vi "FFT_Data_Processing.vi"() -> ()   [LabVIEW 2014]
uses:
  <vilib>/Analysis/baseanly.llb/Mean (DBL).vi
  <vilib>/Analysis/2dsp.llb/Power Spectrum (DBL).vi
  <vilib>/Analysis/2dsp.llb/1D Auto Correlation (DBL).vi
  <vilib>/Analysis/2dsp.llb/Real FFT.vi
  <vilib>/Analysis/2dsp.llb/Cross Power (DBL).vi
  <vilib>/Analysis/2dsp.llb/1D Cross Correlation (DBL).vi
  <vilib>/imath/engines/lvmath2/RunTimeEngine/BuiltInFunctions/win_hamming/NIMS_win_hamming.vi
  <vilib>/imath/engines/lvmath2/RunTimeEngine/BuiltInFunctions/coherence_ms/NIMS_coherence_ms().vi
  <instcachedir>/0/NIMS_coherence_ms()_BC56CBD83C8F45CD8D3E853BABAA39DC.lvgen/NIMS_coherence_ms()_BC56CBD83C8F45CD8D3E853BABAA39DC_000.vi
  <vilib>/imath/engines/lvmath2/RunTimeEngine/ErrorHandling/NIMS_Create Error From Enums.vi
  <vilib>/imath/engines/lvmath2/RunTimeEngine/NodeEndStatement/NIMS_NodeEndStatement_Output.vi
  <instcachedir>/0/NIMS_NodeEndStatement_Output_53EC0D466D134D7ABD903AC30B43404B.lvgen/NIMS_NodeEndStatement_Output_53EC0D466D134D7ABD903AC30B43404B_005.vi
  <vilib>/imath/engines/lvmath2/RunTimeEngine/ErrorHandling/NIMS_Finalize Error.vi
  <vilib>/ptbypt/Signal Generation.llb/Gaussian White Noise PtByPt.vi
  <vilib>/ptbypt/NI_PtbyPt.lvlib
  <vilib>/Simulation/ContinuousLinear/Implementation/NILVSim Transfer Function.llb/SIM Transfer Function (SISO).vi
  <vilib>/Simulation/Implementation/XNodeFramework/SimXNode/SimX.xnode
  <vilib>/Simulation/SignalDisplay/Implementation/NILVSim Time Waveform.llb/SIM Time Waveform (scalar).vi
  <vilib>/Simulation/DataSources/Implementation/NILVSim Pulse Generator.llb/SIM Pulse Generator (scalar).vi
  <vilib>/Simulation/Implementation/Shared/SIMSCR Execution Mode.ctl
  <vilib>/Simulation/Scripting/Companion Diagram/SimConfigNode/_simSolvers.ctl
  <vilib>/Simulation/Scripting/Companion Diagram/SimConfigNode/SimParams.ctl
  <vilib>/Simulation/Scripting/Companion Diagram/SimConfigNode/SimDog.xnode
  <vilib>/Analysis/NI_AALPro.lvlib
  <vilib>/Simulation/Implementation/Shared/SIM Bundle Sim Info.vi
  <vilib>/Simulation/Implementation/Shared/SIM Unbundle Sim Info.vi
  <vilib>/Simulation/Implementation/Shared/NILVSim_FinalizeModel.vi
  <vilib>/Simulation/Implementation/Shared/NILVSim_GetModelError.vi
  <vilib>/Simulation/Implementation/Shared/NILVSim_Initialize.vi
  <vilib>/Simulation/Utility/Implementation/NILVSim Get Time and IsAcceptedStep.vi
  <vilib>/Simulation/Implementation/Shared/NILVSim_Manager.vi
  <vilib>/Simulation/Implementation/Shared/NI_SIM_Implementation.lvlib
  <vilib>/Simulation/Implementation/Shared/NILVSIM_BeginStep.vi
  <vilib>/Simulation/Param Hierarchy/Typedefs/SIMPH Param Control Actions.ctl
  <vilib>/Simulation/Implementation/Shared/NILVSim_ParamChanged.vi
  <vilib>/Utility/error.llb/Clear Errors.vi
  <vilib>/Simulation/Implementation/Shared/SIMSH Read Queue.vi
  <vilib>/Simulation/ContinuousLinear/Implementation/NILVSim Transfer Function.llb/SIM Transfer Function Collector (SISO).vi
  <vilib>/Simulation/ContinuousLinear/Implementation/NILVSim Transfer Function.llb/SIM Transfer Function Distributor (SISO).vi
  <vilib>/Analysis/NI_AALBase.lvlib
panel:
  out "XY Graph":cluster{"X":dbl, "Y":dbl}[](graph)
  out "Coherence":cluster{"f0":dbl, "df":dbl, "magnitude":dbl[]}(graph)={"f0"=0.0, "df"=5.029169181251257, "magnitude"=array[24855 elements]}
  out "size(s)":i32=24856
  in  "INA Resistance":dbl=1000.0
  out "array":dbl[][](array[numeric])
  in  "file path (use dialog)":path=path "D:/Academic_Gaduate/Course/2016 Spring/2.131/Project/MyRIO/DAQ and Actuation DIO Stochastic Double Input 125kHz differential measurement and system ID with Bode Plot Analysis/04212016/RC/BinaryStochastic/042116_RC_Stochastic_4.csv"
  out "Phase spectrum":cluster{"f0":dbl, "df":dbl, "phase":dbl[]}(graph)={"f0"=0.0, "df"=5.029169181251257, "phase"=array[24855 elements]}
  out "Amplitude spectrum":cluster{"f0":dbl, "df":dbl, "magnitude":dbl[]}(graph)={"f0"=0.0, "df"=5.029169181251257, "magnitude"=array[24855 elements]}
  in  "Sample_Frequency (Hz)":dbl=125000.0
  out "Waveform Chart":waveform(dbl)(graph)={"t0"=timestamp(0.01 s since 1904-01-01), "dt"=1.0, "Y"=[1.8810764409104788]}
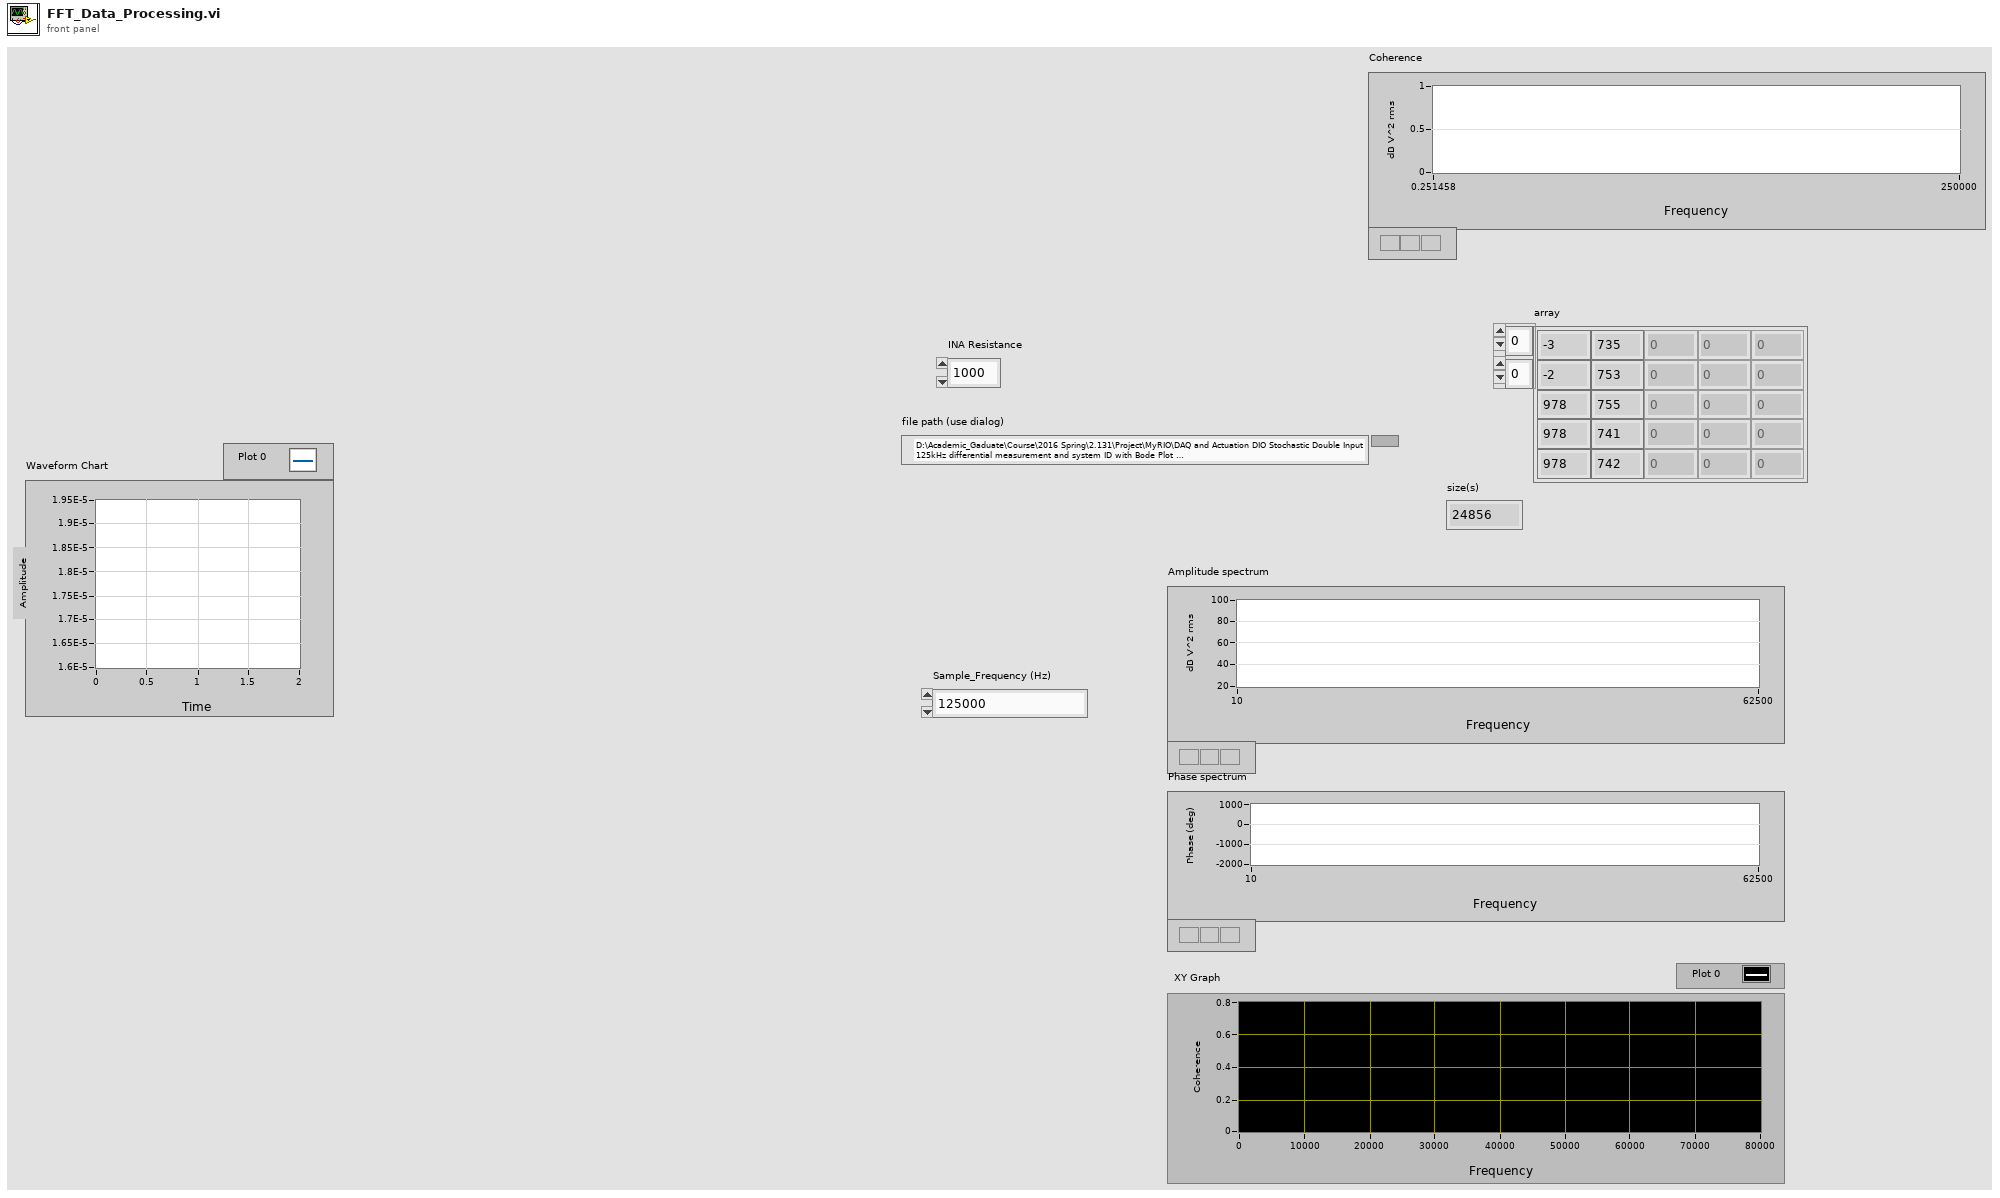
[diagram p1: front panel]
types:
  T1 = enum16{"open", "replace", "create", "open or create", "replace or create", "replace or create with confirmation"}
  T2 = typedef "SIMSCR Execution Mode.ctl" = enum16{"Simulate to Completion", "Single Time-Step Simulation (Fixed Step Only)"}
  T3 = typedef "SIMPH Param Control Actions.ctl" = enum16{"get params", "set params"}
  T4 = typedef "SimParams.ctl" = cluster{"Initial Time (s)":dbl, "Final Time (s)":dbl, "Step Size (s)":dbl, "ODE Solver":T5, "Minimum Step Size (s)":dbl, "Maximum Step Size (s)":dbl, "Relative Tolerance":dbl, "Absolute Tolerance":dbl, "Software Timing":bool, "Initial Step Size (s)":dbl, "Automatic Fixed Step Size?":bool, "Automatic Discrete Step Size?":bool, "Discrete Step Size (s)":dbl, "Calculate using Time Step":bool, "Solver Wired?":bool, "Prev.Frm.Expected End":u64, "Prev.Frm.Actual End":u64, "Prev.Frm.Finished Late?":bool, "Prev.Iter.Expected End":u64, "Prev.Iter.Actual End":u64, "Prev.Iter.Finished Late?":bool, "Expected Iteration Start":u64, "Actual Iteration Start":u64, "Expected Frame Start":u64, "Actual Frame Start":u64, "Source Name":string, "Name":string, "Period":i64, "Deadline":i64, "Offset":i64, "Start":i64, "Priority":i32, "Timeout":i32, "Processor":i32, "Mode":enum32{"No Change", "Process missed periods, maintain original phase", "Discard missed periods, maintain original phase", "Process missed periods, ignore original phase", "Discard missed periods, ignore original phase"}, "Wakeup reason":enum32{"Normal", "Aborted", "Asynchronous wakeup", "Timing source error", "Timed loop error", "Timeout"}, "Error":errorcluster, "Source Type":string, "Secondary Source Type":string, "Global End Time":u64, "Global Start Time":u64, "Full Solver Reset":bool, "Execution Mode":T2, "Nan/Inf Check":bool, "Custom Solver Library":string, "Solver Is Variable":bool, "custom solver name":string, "Signal Collection Decimation":u32}
  T5 = typedef "_simSolvers.ctl" = enum16{"Runge-Kutta 1 (Euler)", "Runge-Kutta 2", "Runge-Kutta 3", "Runge-Kutta 4", "Runge-Kutta 23 (variable)", "Runge-Kutta 45 (variable)", "BDF (variable)", "Adams-Moulton (variable)", "Rosenbrock (variable)", "Discrete States Only", "SDIRK 4 (variable)", "Radau 5 (variable)", "Radau 9 (variable)", "Radau 13 (variable)", "Radau [Variable Order] (variable)", "Gear's Method (variable)", "Linearizer", "State Query", "Trim Eval", "Custom Solver"}
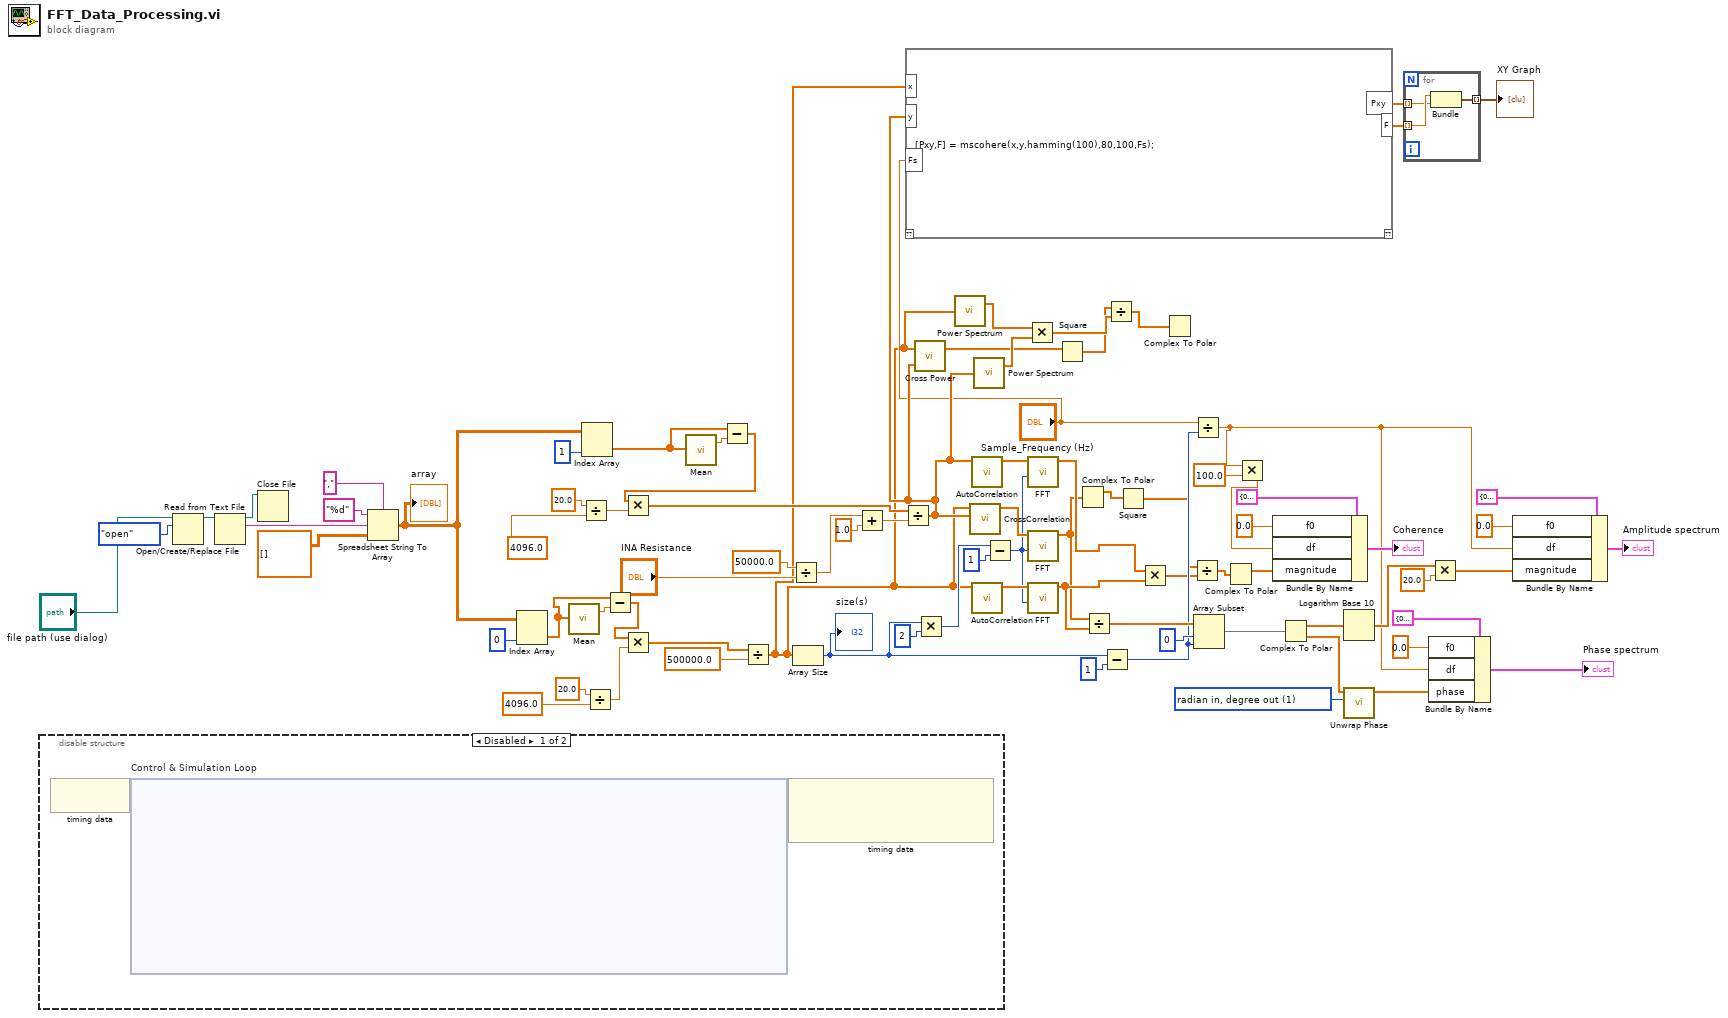
[diagram p0: block diagram]
diagram:
  w39 = 1 items=["radian in, radian out", "radian in, degree out", "degree in, degree out", "degree in, radian out"] ("phase unit")
  n1 = disable-structure shown="Disabled" {
    frame Disabled {
      n2 = node-c288() -> (w85:variant)  [unwired: 1 in]
      n3 = node-c254 "Control & Simulation Loop"(w85) -> (w84:variant)
      n4 = node-c288(w84) -> ()  [unwired: 3 out]
    }
    frame Enabled {
    }
  }
  n5 = Open/Create/Replace File(file path (use dialog)="file path (use dialog)", operation (0:open)=T1."open") -> (refnum out=w81:refnum<file>)  [unwired: 4 in, 2 out]
  n6 = Read from Text File(file (use dialog)=w81) -> (refnum out=w76:refnum<file>, text=w79:string)  [unwired: 3 in, 2 out]
  n7 = Close File(refnum=w76) -> ()  [unwired: 1 in, 2 out]
  n8 = Spreadsheet String To Array(delimiter (Tab)=",", format string="%d", spreadsheet string=w79, array type (2D Dbl)=dbl[][] []) -> (array=w23:dbl[][])
  "array" <- w23
  n9 = Index Array(array=w23, index (col)=0 ("disabled index (col)")) -> (element=w19:dbl[])  [unwired: 1 in]
  n10 = call-poly <vilib>:"Mean.vi"("X"=w19) -> ("mean"=w20:dbl)  [unwired: 1 out]
  n11 = Divide(x=20.0, y=4096.0) -> (x/y=w52:dbl)
  n12 = Index Array(array=w23, index (col)=1 ("disabled index (col)")) -> (element=w22:dbl[])  [unwired: 1 in]
  n13 = Divide(x=20.0, y=4096.0) -> (x/y=w45:dbl)
  n14 = Subtract(x=w19, y=w20) -> (x-y=w18:dbl[])
  n15 = Multiply(x=w18, y=w45) -> (x*y=w31:dbl[])
  n16 = call-poly <vilib>:"Mean.vi"("X"=w22) -> ("mean"=w21:dbl)  [unwired: 1 out]
  n17 = Subtract(x=w22, y=w21) -> (x-y=w17:dbl[])
  n18 = Multiply(x=w17, y=w52) -> (x*y=w30:dbl[])
  n19 = Divide(x=w31, y=500000.0 ("x")) -> (x/y=w8:dbl[])
  n20 = Divide(x=50000.0, y="INA Resistance") -> (x/y=w50:dbl)
  n21 = Array Size(array=w8) -> (size(s)=w61:i32)
  "size(s)" <- w61
  n22 = Add(x=w50, y=1.0) -> (x+y=w41:dbl)
  n23 = Divide(x=w30, y=w41) -> (x/y=w10:dbl[])
  n24 = mathscript code="[Pxy,F] = mscohere(x,y,hamming(100),80,100,Fs);"("x"=w8, "y"=w10, "Fs"="Sample_Frequency (Hz)") -> ("Pxy"=w1:dbl[], "F"=w2:dbl[])  [unwired: 1 in, 1 out]
  n25 = call-poly <vilib>:"Cross Power.vi"("Y"=w10, "X"=w8) -> ("Sxy"=w11:cdb[])  [unwired: 1 out]
  n26 = Multiply(x=w61, y=2) -> (x*y=w72:i32)
  n27 = call-poly <vilib>:"Power Spectrum.vi"("X"=w8) -> ("Power Spectrum"=w16:dbl[])  [unwired: 1 out]
  n28 = call-poly <vilib>:"CrossCorrelation.vi"("Y"=w10, "X"=w8) -> ("Rxy"=w74:dbl[])  [unwired: 8 in, 1 out]
  n29 = call-poly <vilib>:"AutoCorrelation.vi"("X"=w10) -> ("Rxx"=w37:dbl[])  [unwired: 9 in, 1 out]
  n30 = call-poly <vilib>:"AutoCorrelation.vi"("X"=w8) -> ("Rxx"=w75:dbl[])  [unwired: 9 in, 1 out]
  n31 = call-poly <vilib>:"Power Spectrum.vi"("X"=w10) -> ("Power Spectrum"=w15:dbl[])  [unwired: 1 out]
  n32 = Subtract(x=w72, y=1) -> (x-y=w36:i32)
  n33 = Multiply(x=w16, y=w15) -> (x*y=w14:dbl[])
  n34 = call-poly <vilib>:"FFT.vi"("FFT size"=w36, "X"=w37) -> ("FFT {X}"=w27:cdb[])  [unwired: 8 in, 1 out]
  n35 = call-poly <vilib>:"FFT.vi"("FFT size"=w36, "X"=w74) -> ("FFT {X}"=w24:cdb[])  [unwired: 8 in, 1 out]
  n36 = call-poly <vilib>:"FFT.vi"("FFT size"=w36, "X"=w75) -> ("FFT {X}"=w26:cdb[])  [unwired: 8 in, 1 out]
  n37 = Square(x=w11) -> (x^2=w12:cdb[])
  n38 = Complex To Polar(r * e^(i*theta)=w24) -> (r=w25:dbl[])  [unwired: 1 out]
  n39 = Divide(x=w24, y=w26) -> (x/y=w63:cdb[])
  n40 = Subtract(x=w61, y=1) -> (x-y=w58:i32)
  n41 = Divide(x=w12, y=w14) -> (x/y=w13:cdb[])
  n42 = Square(x=w25) -> (x^2=w28:dbl[])
  n43 = Multiply(x=w27, y=w26) -> (x*y=w33:cdb[])
  n44 = Complex To Polar(r * e^(i*theta)=w13) -> ()  [unwired: 2 out]
  n45 = Divide(x=w28, y=w33) -> (x/y=w29:cdb[])
  n46 = Divide(x="Sample_Frequency (Hz)", y=w58) -> (x/y=w7:dbl)
  n47 = Array Subset(array=w63, index=0, length=w58) -> (w64:cdb[])
  n48 = Complex To Polar(r * e^(i*theta)=w29) -> (r=w4:dbl[])  [unwired: 1 out]
  n49 = Multiply(x=w7, y=100.0) -> (x*y=w5:dbl)
  n50 = Bundle By Name(cluster=cluster{"f0":dbl, "df":dbl, "magnitude":dbl[]} {"f0"=0.0, "df"=0.0, "magnitude"=[]} ("Amplitude spectrum"), "f0"=0.0, "df"=w5, "magnitude"=w4) -> (→"Coherence":cluster{"f0":dbl, "df":dbl, "magnitude":dbl[]})
  n51 = Complex To Polar(r * e^(i*theta)=w64) -> (r=w60:dbl[], theta=w38:dbl[])
  n52 = Logarithm Base 10(1:w60) -> (0:w68:dbl[])
  n53 = call <vilib>:"Unwrap Phase.vi"("phase unit"=w39, "Phase"=w38) -> ("Unwrapped Phase"=w40:dbl[])  [unwired: 8 in, 1 out]
  n54 = for {
    tunnel: w2 -> [w406] mode=indexing
    tunnel: w1 -> [w405] mode=indexing
    tunnel: [w404] -> w3 mode=indexing
    n55 = Bundle(w406, w405) -> (w404:cluster{dbl, dbl})  [unwired: 1 in]
  }
  "XY Graph" <- w3
  n56 = Bundle By Name(cluster=cluster{"f0":dbl, "df":dbl, "phase":dbl[]} {"f0"=0.0, "df"=0.0, "phase"=[0.0, -31.46771497568485, -28.75800712836132, -41.40521112388251, -28.23254003958854, -10.307643755414622, -48.402035704012796, -54.988080356169355, -6.260155572788149, -114.48865953158258, 8.840814305252367, -81.75181328535328, 2.5045447437835056, -4.4432479279741095, -91.23410525561975, 31.80581741631602, -114.44832858997734, -27.80131859077831, -99.25569904439564, -30.088844331129934, -103.06596414735802, -66.66233183584428, 12.455917853016478, 109.28759197945335, -66.14168263333863, -144.83425351569642, 51.71723004569318, -59.12936901186461, -59.94315211957277, -44.52651345174281, -83.39567725724885, -88.80210274367009, 173.64945828897015, -22.022991001879543, -176.90163746313618, -45.43423776031069, -174.56084625229602, 23.97985521334657, -111.39703590450088, -88.75411195664891, 17.490204367239716, -109.71720216205237, 15.903183296946878, -63.74675570783637, -76.38848380866358, 90.4171618729539, -67.70206212228267, 173.17746062348021, -63.34328741918001, 97.88702687250597, -26.830346465652713, -178.56862486837178, -28.233947423969404, -69.71520075870326, -93.38491152339505, 172.31861385368967, -24.72816138371724, -158.6603632884339, -63.92637331120567, 25.979182283576865, -176.178680883384, -54.992745526133994, 154.66292784768336, -21.75898247362432, 147.62448353052594, -48.4012168873971, 173.61513877249942, -91.40498135572582, -29.27842403446698, -90.12818047003235, 44.89492509568193, -85.02569711983062, -161.62807827258007, -30.33210234328775, -167.38943949322578, 17.714982838532073, 128.95801741205386, -67.90830100247624, 133.7770774630165, -28.626976629449626, -63.62310170383254, -117.87464062810677, 81.94531443559661, -93.09760124996781, 23.909644860719627, -101.32638644807278, -24.510873351315627, -168.41200063244855, -72.35935696130369, -155.28973739698282, -17.847314598481347, 78.21905993530349, -75.2179881300336, 158.254123483706, -113.64472897818374, -7.605633196806257, -179.31194749940937, -31.704382462216028, 176.59993683257554, -3.9100568867706125, -175.3215455037979, -37.06483139906273, -143.58448093876837, 20.571245493011833, -118.99832924113697, -96.78723400578556, -60.086953107243204, 122.97366891032519, -45.543749408235314, -91.64436597307613, 27.874487865472883, -44.86713542183372, -178.07594038380435, -86.92786166047328, 82.4094513217639, -78.34921684511612, -173.92693798878386, 102.4715615364932, -33.202770362216675, -119.88125106432467, 27.96070642572587, -143.51766607705275, -110.53171785865658, 14.030389804595977, -14.364430460296093, -121.02086313650614, 41.55311803721051, -82.14295365670695, 4.975296548772393, -146.7149096680376, -101.59304285295177, 29.849633712272396, -82.48816912553207, -149.48005476874508, 17.8777224533454, -153.22017067339883, -55.88267286162645, -73.12223389390026, -177.0689123580233, -101.71777995720713, -19.5987345915357, 48.39071628315272, -104.51560193133216, 106.24875412055499, -64.62181776044855, -152.49158868871936, 90.50578375571689, -110.23177544712142, 178.7743822962101, 8.933446493462752, -117.43777414097968, 33.78573575385322, 3.753644677644808, -133.54790142199468, 155.06753756966313, 1.313093243393488, -135.93501009935378, 102.88813110897146, -65.0985044001864, -22.667258074295468, 139.20059133429496, -50.73701255959797, 169.65584439562346, -4.395964236758193, -65.67336673335154, 95.38893308207317, -151.4067275831482, -135.1595759134875, -50.630333757584644, 86.38052475049209, -105.4818844884823, 48.68364954626779, -63.32067960398621, 152.87921036982615, 11.833828912216703, -14.298996026707998, -153.77260213733103, -43.14750001054217, 59.32361441752411, -131.55695844776793, -58.17994776721444, 70.44010783175709, -128.00748777563172, -68.53969421568672, -21.430548261334962, 132.6995122419159, -57.382207495062104, 104.60385375657543, 176.2681159822832, -12.528130482428411, -113.88004350080426, 6.718207285255911, -158.558628085825, -74.33498613287863, 83.3039064212861, -159.12090829011342, 10.554276562274639, -75.93691675536499, 53.72426810131386, -147.92326776688313, 42.16756652088333, -110.59744086394932, 13.00099316823571, 42.89530864726003, -78.5100056583534, -14.864119179247732, 151.771235214809, -53.33854934192464, -50.18504546090332, -78.10915320757155, 107.61492267174592, -41.731323391150696, -171.9549311336031, -31.909487386903535, -54.76941049884478, 161.99647147822193, -23.644807465324686, -139.42463002301935, 48.18016831507575, -137.63420984995042, 12.858622069483772, -144.83283655524738, -78.58801072388744, 56.23414488656744, -82.52800501693756, 165.1339518127335, 30.985754421181294, -50.87159030515992, -108.7703977965099, 104.96572974047947, -45.2937013625406, -108.84268401885568, 44.80515131574169, -139.81653610936894, -5.854579467043601, 139.24625549981425, -34.43047469570014, -130.57782005611404, -75.90546203446466, 76.71414237862456, -115.33869977557293, -152.1695207386769, 23.916191636708742, -157.80987721359594, -7.3317827307557675, 118.03670607456142, -122.24723240808913, 7.45872793350562, -40.91520539379452, 126.433151740827, -66.45542530364317, 111.57432009746935, -72.44942344083017, -177.4506210892957, -98.91073477511371, -7.729660477553103, 10.465818868467291, -85.6936671592382, -81.63472484446946, -142.59977661658678, 128.460132193279, -38.475073345298455, -67.30940359671469, 123.49482022783103, -97.1053140060935, 145.19216903060635, 19.599574149358055, 86.71319792618822, -59.42600601366192, 144.78547374608254, -0.14154390010495188, -31.99696885455758, -95.14990183095408, 17.55567657493523, -114.4051716245541, 123.83652692238601, -54.112354263827676, 111.56127409377314, -96.23472855569044, -164.82585042487696, -5.170563653506037, -152.92260427891915, -144.945554637376, 4.847235795070112, -119.10529254609949, 125.58380441248624, -63.22633423069135, 16.491596036524914, -169.19469396356925, -59.49742518985056, 99.33906473700418, -83.19230064604379, 94.70172496456746, -69.26753585553224, 93.20284400521376, -149.19174515783365, 32.644347404502724, -144.99653166541907, -5.748775767562918, 132.46944910894436, -70.188539813744, -175.15797843215728, -18.781631461778034, 139.2296455769892, -45.83812731645386, 159.7977626761071, -9.006363901405047, 148.21713714850534, -100.8278607774186, 55.930164359566405, -158.55075386155477, -103.64878607543045, -47.70206737703835, -65.34411503659574, 67.87094437951615, -154.64047195169766, 97.88783811393293, -5.57745461676379, -78.1709697035549, 78.52481788767172, 161.5334038052565, -109.8413047486903, 71.77211881090538, -4.575980521272304, -133.59202718799017, 61.733256861048496, 178.73417565413922, -47.53771825336581, 125.45827259728232, -97.1902841273301, 52.950131640632364, -154.25843315518011, 5.8136678258338845, -155.26807894125346, -51.157307142112785, 99.78819729052276, -48.97948721442834, 169.6472766422358, -117.99599455441421, 25.708792715303733, 131.97176948195855, -64.40284134065979, 111.90384579625118, -127.68827211261325, -77.79968188970696, 43.89611166074449, -160.45284620783127, 8.44734072748546, -149.78104520145075, -77.22735970987173, 159.98715516082572, -89.99063430205264, 45.70732002040879, -139.86300077763389, -6.566845107941335, 178.30876547862576, -22.561851211410573, 37.55133985052249, -149.05052759820148, -29.6953915669966, 95.88142220084387, -101.30091321782635, 23.223671482431147, -157.61569681073925, 32.07479172229752, -71.3688731058624, 2.5795540168955897, 120.05824105976018, -95.05769691572468, 37.51344432680482, -121.41122349093216, -142.04667587013134, 45.927259881274615, -134.5453172929541, 33.96968894493717, 153.058526546883, -140.03677728629194, 3.5646310942392696, -175.37291939786292, 14.115882878139795, -156.173477913963, -70.16579453905345, 91.56497193006136, -77.36117907923929, 59.233660597809425, -127.4719648111601, 56.51477730558104, -84.79620262857178, 86.58630420746188, -118.28259178761235, 22.600459669840806, 146.04464592728684, -77.89681873325401, -5.689349256760081, 177.24762803403777, -67.73763403578465, -1.8103440796276928, -115.0305743613975, 42.78528548717108, -106.57160168656428, 101.99012391694329, -102.41599801509702, 49.34066109247137, 178.44665732631697, -61.34206176169528, 132.87965238205607, -11.546056273837774, -125.65619450370565, 54.12229834647187, -127.60567202299247, 48.993493963204884, -16.604257356824057, -173.03075984094417, -47.372369968303495, 46.82445661446543, 68.31108839735339, 76.53022405615046, -159.4911598984052, 36.484166933763284, -47.776958039264834, 152.2068219538879, -69.4577862169963, 23.72800166288421, 151.48388845297458, -16.493785662288833, -171.7401814752173, -64.656079915525, -56.13125155943886, 82.01996288505002, -63.94387574731906, 124.71550967915313, -104.95295949349935, -67.38813885713685, 77.12067398170372, -101.33147779856687, 99.31134042143898, -64.55196472267788, -151.67999889218746, 113.13764572404774, -36.53419971497588, -134.1711272925018, 71.0322618140203, -163.46692161183003, -130.37776991970134, 58.37272802003515, -107.62472868622736, 92.95279272623449, -49.150748419198734, 159.36012917745043, 55.28737975676292, -110.16360848814493, -53.79860569519096, 104.49602190989943, 148.55577400818933, -30.020328942202788, -68.77381027418048, -42.15810867554653, 124.2170657880268, -86.95369614934374, 44.99512130882773, 177.32845100229312, -52.64196228170846, 46.20102763955148, -108.80445041232439, 62.10585572867235, -102.53934126921365, 145.9677583834663, -87.72193055370626, 7.430962421708717, 172.95218029826705, 4.4222030934162095, -131.33811798336814, 37.479163647581316, 137.83109311522614, -34.772558001913914, 152.95764683962005, -26.945111117281396, 166.68720416268573, -28.35898721082636, -102.96758495536596, 99.62582554177011, -81.23530180181987, 46.95581407891729, -125.39186806017632, 141.14774219662723, -65.91933405996008, 124.5369717528866, 112.16827006625896, -52.174323660626484, 130.56766513060325, -92.17901272631585, -99.80861309109997, -15.580125933333163, 178.68459291382678, 65.85001986602701, -85.62453959075624, 80.16771494845275, -63.09056610855369, -22.22041093173988, 142.374831558324, -22.723043570811264, 179.6131973929219, 1.0719245177840404, -88.1651047885446, 117.3162732148612, -60.235562901182256, -107.97892141496881, 162.13789603953347, 12.79775668263484, -159.941273163866, -112.3033138485895, -6.702876591119159, -175.53346605334087, -32.7521632120629, 148.57881181169574, -11.417752403481312, -169.89475358248, -33.20930187301011, 82.27334674193816, 172.04980593620093, -122.82110283025958, -42.916824763589396, 46.67338200369259, -155.2949042573867, -105.63553113653434, -107.62874242849799, 11.775202677368716, -171.23287115203678, -2.029325683277578, -162.5560667916255, 73.31010367618042, -107.93952835877826, -83.0493564353863, 52.09254527340971, -143.1028799072984, 53.765912683226226, -34.19495582188307, -117.75357133516779, 31.834257499681126, -140.93286631533525, 20.285152783977193, -162.04195864800806, 153.64371771682758, -73.66007185930609, 15.963436915003053, -171.21157098983684, -47.68895068390904, 66.4135578918687, 174.73664348470854, -46.579508638827356, 106.03859109730527, -109.91539448636465, 39.172417305631974, 145.77979102715958, -9.962680136496868, -164.42924385477494, -144.44561580277627, -69.78123459385885, -113.22071531978678, 1.218258742126064, 143.16141050902604, -157.77775989154455, -30.270285893319095, 166.15106846550387, -45.34197099655759, 137.05342066451018, 20.241780198571846, -102.77142543056473, 31.439785015283583, -121.94168892212197, 143.20819621702185, -19.50689927100417, -172.02714961369415, 14.333717594969812, -174.54550977736082, -38.23299518978718, -26.566119797522497, 145.54151457275842, -27.851441052904736, -163.1321157748263, 75.3014631451511, -94.74166019476999, 37.075911773395255, 155.54222543194072, -98.9395351512745, 148.13703747510186, -17.54789487058411, 143.79080232675827, -82.71301752835367, 71.3821044984081, -124.21247549991963, -1.6409856573868462, 19.6700330708455, 160.14775353560006, -16.49430253911016, -164.78180265396531, 12.760891558196134, -179.47420233424083, -5.793119973627547, 69.40140401989008, -85.35709611715286, 120.10014940793037, -104.09159686676787, 26.31025850963576, -83.18524249721266, -179.06877555105402, 71.26471876869424, -65.84400382413854, 19.518368314758515, 154.98160428075326, -39.27619259227029, 163.50923755813903, -50.03350589385845, -9.115898207634226, 130.84824117370394, -46.68826854993543, -148.71498865685814, -22.5834873291525, 132.6178627343492, -134.46027090254492, -2.8014924912677923, 2.4602588300456407, -20.736466264500084, -130.69158165429175, 150.66416663985305, -11.018068033122065, 171.6304217452683, -96.58990485321286, 77.83444641407394, -99.09283298242498, 88.80014570919934, -40.586998724210204, -35.179264249983795, 160.7340227956574, -6.810605241887145, -139.76389074792675, 61.4695137232016, 21.189936050034103, -98.82360269013745, 116.59527939088214, -8.355189026823824, 175.8100810017669, -8.629108482243616, -173.90491830172104, -79.85592225607972, 87.32016128248391, -91.81291748729721, -13.435477477820484, 96.50857130191405, -109.38180407495078, 33.06042963793669, 162.2011521762079, -117.94163565196628, -4.833287709282053, -62.12189719388706, 116.03937464806818, -57.917706915940535, 149.82527299038165, -51.82821745375959, 122.61039417676135, -44.556770160055926, -178.79931798390376, 73.21959964459208, -49.68220726056265, -88.4753258698242, 85.97647885149128, -38.29177733636641, -143.88884710240126, 5.282625504869, 141.10625269184, -57.50253327360124, 39.18691565225554, -159.6754196513465, -116.14617655830526, 95.22297266469835, -144.2484002418386, 28.899643887893554, -144.2272853862776, -37.74225611166511, 102.20586557689614, -59.82479773715672, 127.04189962515147, -46.24791124113113, 68.08629766481732, -156.7578294816097, -11.434921889037966, -162.7636201167861, 65.9875644978628, -34.46832773201904, -78.56948038746317, -6.341337929151649, -108.67685939124134, -106.89313197435935, 86.38952053728252, -82.93911771001973, 173.25389098385997, 67.40056048245822, -125.26619173900407, -37.805267152913395, -175.16220300153662, -140.71414280919208, 24.3021970024091, -150.81559287743767, 61.64820799188565, -135.28671942766917, 52.632055272904026, -89.42932587679499, 98.47854234743062, -39.87945695164611, -162.66519730541248, 11.68692118129435, -166.08307632599565, -88.98536844861681, 87.7653832187781, -59.430681173676724, 107.1788677654589, -87.82119051152033, 51.711884791693265, -178.07871544746556, 37.41838157670529, -55.35611367871979, -84.61570240600459, 94.65796995336078, -129.98746807541917, 58.335236715745765, -99.00946937428698, -27.388117599098656, 157.22388234666346, 72.24371871312997, -147.39896486209406, -132.6777473905325, -31.25385142571185, 74.26515240712175, -84.67039004635154, 94.80636631950513, -174.6516234468396, -170.3480501081504, -48.02777153805316, 51.75317164614029, -91.701517555401, 133.0172297974163, -7.30159849250651, -113.17171907810842, 44.91847253132216, -101.68955446502213, -112.83910396609542, 76.41050489240513, -96.71151005959905, 62.37966193166177, 174.59527102428734, -74.50503041737309, 102.74242740569944, -167.43185591844207, -28.974517625091067, 114.03751275726806, -52.52542778132872, 140.60970417095436, -43.560106659883395, 148.19389046654692, 62.03454906051373, -37.963677576846045, 154.55973613044287, 146.4805228355848, -16.955183383517827, 160.5658961892464, 41.884605965508264, -102.22531021640862, 66.33884226578459, 125.35537253171245, -93.07124847733196, 43.603115837203596, -35.825264703512545, -134.75332606919338, 140.3915945396924, -170.58539119057713, -4.3555387719877405, 166.02689974489226, -173.60083831016271, -0.12867793207221537, -164.76794171616692, 39.46321438891706, -71.26099387456847, 117.49796589596059, -32.12016123027836, 7.625896306543184, -151.83905484477293, -48.434939537281075, 53.64831087302935, -93.18411966205646, -98.36993493084799, 119.87917242870013, -108.55893117369165, -81.9910561163668, 95.0089679392402, -72.73671350427458, -14.702075420706603, 144.29025842674645, 3.0096227078141595, 174.39608030714825, -47.32134892884564, 130.1200593091527, 3.010297210957817, -149.96378770274794, 5.15648604979302, -131.00767475137724, -139.2648166197183, 51.05469049011057, 137.7627910319741, -129.56436731345153, -4.398610626420822, -128.85975701865624, 172.0314351621999, 19.536121307586072, -128.33535280968172, 115.03643800205525, -167.4008694494514, -99.78729461742101, 2.1618823895867507, 175.86714720509178, 27.870601656544217, -134.23437033976293, 61.752379570873074, -58.764272188723105, 140.50940594389758, 17.401790900348622, -76.88446792601037, 112.93800811739614, -74.47023687960714, 57.75177664789759, -135.33399721576845, -4.171499467230711, 158.58563404735605, 0.3753823843596019, -124.364687997409, -71.42039127455385, 89.7699642964547, -61.78524015886245, 139.76552443283884, -48.05344181609611, 172.2204000780463, 6.5441568360572555, -161.357014987678, -163.859193026889, 31.148918252059225, -74.63094220037475, 54.449483825565146, -141.07611084637665, -59.928523683736344, -111.59721137682088, 136.18591667878417, 51.20836380129699, -102.00998276251163, 69.38881272956878, -6.650584423835163, -119.84758918182608, -171.28476431719838, 31.745429699844387, -146.88562824741777, -41.455445941199955, 53.61648403891242, -83.30618114791412, 174.65974179855394, 98.65615679714519, -35.27670632618104, 94.2201132403794, -155.93415721486912, -6.581542390692745, -179.32672267917255, 175.13750093955665, -14.377608913808187, 148.30243299082807, -75.77067841132367, 38.9797740122615, -132.1587412992525, 106.49646205369946, 8.407250852124852, -35.496741621256454, -173.13138141404895, -15.555504023221577, -41.09548969322256, 103.51834305585722, -76.63858633555844, 83.08988233557466, -104.31389048078786, 152.10523290311446, 24.12399022599241, -111.12207877005906, 78.26259707356425, -112.02416060399644, 15.314106421968939, 101.82627173313676, -93.85166587574152, -78.05401638398496, 80.07712418944736, -124.77812823558038, 35.24366770793687, -175.3845889000318, -132.36572514301386, 40.5756213070226, -156.20187378885308, 171.9056817310974, -39.56045326497815, -168.07294285346202, 69.84033971188616, -128.70404232383888, 55.7018856169047, -106.91461481830608, 61.33433465707653, -79.25612475595284, 120.3157571372352, -31.727767728482117, -131.03860078296557, 52.30500145215631, -22.159778917101875, 47.784773735495726, -167.58098485630725, 61.19805538687596, -97.43659050196452, 172.61620968167725, 79.22607520811626, -95.95857423816624, 66.45261522120416, -84.99681059301679, 90.93092605365476, -109.87924739570839, 81.26444224879198, -48.34416826511803, -64.58180703086579, 113.04578180460125, -144.14356122698217, -80.56638369325132, 127.20020340250167, -15.790373595853024, -157.42916772921131, 21.76267915547008, -136.17702934094277, 50.2139369865897, -154.41573695824312, -164.69841826446915, -40.1461390295112, 82.87549806880557, -150.8276598487717, -155.32164437089392, 29.07811399210879, -131.55644653954394, 46.5886125420891, 115.534594263016, -170.74352806061225, -178.07643257281725, -33.8592969908437, 168.5947907083288, 20.449565770055152, -75.94060482167131, 158.8245430480659, -112.66598853349507, 38.89086498336261, -166.79863316540067, -6.517461844467805, 172.40336008682024, -108.48333231469148, 103.0077494423459, -64.50414566315867, -136.18318082417616, 121.90959062406351, 17.62808828196523, -130.10130419048264, -51.59008466077416, 105.37193135664373, -13.657510537797231, 173.278254098405, -48.281838423108304, 92.6388600471226, -146.71711678618286, -67.47884374368712, 29.239815840975087, -160.28233925130934, 0.8888929126289344, -102.01731279509282, 154.70709695376993, 38.58666867618779, -111.13600269589034, 100.34335245842009, -34.71662325705039, -172.54277250457474, 6.955855118340482, -132.12785554193343, 29.157041764966515, -170.8670063921851, -11.913089917779487, 146.84381016637272, -81.34652736348627, 115.26904866809885, -36.1622508877769, 7.692666299287185, -105.92571691415164, 71.34585535941753, 154.26619763328253, -114.78408569593822, 37.29958128822877, -86.67582541117214, 120.29445840382922, -20.760740585816038, -96.02829573330683, -163.5243218673722, 12.34584961728268, -122.09167019104686, 44.099190833483036, -137.98280780976518, 13.02176601697639, 175.3128113036764, -73.80936690660296, 57.539304281570644, -103.18082673162364, 62.685482872660685, -140.1758319397973, 23.951905777259654, -140.56556771001314, -3.503972735778517, 8.401638219489543, -177.55753622028843, -42.2531169815855, 80.60614179910885, -97.8381137940205, -141.70635496568957, -33.90917696768902, 55.5536770928396, 140.7268769508222, -141.05613335468698, 169.02167705315165, 47.86101633636791, -63.87780954729518, 146.22912277482766, -45.517548029819814, 157.62427693501417, -146.3763730069418, 19.309334210416754, -162.66139438135335, 110.1156921199843, 0.4058277877374209, -158.93678076518034, 65.12622208937746, -48.13105936849473, -90.61693266589735, 110.3684208516205, -47.55892328814662, 99.13307845411279, -118.35652113019763, 86.7725094101466, -50.675095420006926, 36.44276216000854, -70.41582180690077, -148.76165988132578, 102.01189215831464, 90.5184122875831, -39.26716389274115, 140.49553248572906, -9.73532581901628, -138.06187576641122, 92.5513845826085, -13.104884407640691, -67.57137392081415, -128.24056863758096, 67.158018656186, 55.64923214058838, -61.22606891718426, -37.73999045685493, 144.64419613044365, -43.43982326787414, 151.58814064931013, -30.160983692261773, 174.92741734752164, -32.57593716478941, 132.3070887939625, -84.07963723133689, -14.010764751987635, -147.3930895585615, 6.234462628506151, -175.94338025911424, -15.244944229533209, 61.01046970901816, -148.76854742908296, 22.95297181907012, 167.85578376026874, 165.56024240810922, -106.55067829350371, 54.114956495601966, -124.06736579169039, -20.928595265098167, 145.76043687026737, -20.64649020005843, 142.82395115961256, -112.2742215801115, 25.605265591621396, -129.35562247924895, 77.0850466752252, -62.533685569094594, 121.88645034810256, -118.69071498553743, 19.897521078087657, -144.1895892757996, 42.077199094355805, -97.79253359679633, 147.29708449465124, 6.140214960534181, -150.4544838759599, 1.079354270382953, 75.5755587756743, -23.75984705987529, 128.81648317661876, -105.53984014794835, -64.55489273500467, 91.24698990320063, -19.636650666370766, 173.22401919791056, 25.74750306003994, -132.0396172291538, 160.36632424735924, -36.600952870697974, 148.93903947158813, 19.92946182742798, -68.40556641566, 122.73531129611327, -84.68677427453405, -65.37331364093983, -143.74261844943265, 37.731442060816946, -161.25792922100717, -63.128693260199995, 120.56153179564413, -51.31228196792734, 104.88172590535794, -94.9143885366642, 65.51696039694097, -147.2823799294896, -40.31066244255004, 65.43115316589335, -136.62943074955518, 9.185584203648206, -78.95689771503193, -84.58118515457805, -169.21389367455365, -0.19782341454660116, 108.54764039668675, -60.6311399206834, 147.01842057658908, 19.53110810627237, -148.5620542429298, 50.57930748032758, 25.79535476584446, -120.50817274124576, 54.257018576717755, 112.7340766697778, -68.7410594512242, -118.03055410363083, 89.44728816500704, -47.22049903002262, 141.51976662279975, -85.66669296215572, 144.93707593344953, 3.6732526693273, -168.2518999626591, 3.101742027927127, -97.67755303452523, 147.87157232094745, -108.239315195582, 92.18943746392112, -75.1085500661009, -50.29542452383882, 79.7294159676927, -136.08761793430557, -11.454348805669973, 40.59089972858454, -177.9700989847409, -56.14023059896699, 95.2943464381373, -24.14447012536165, -150.4496205572934, -46.20633653055355, 67.54565882713658, -108.7685483792471, 65.77185813927026, 18.904590499594097, -139.73064081969142, 16.48941570477792, -141.95959374959625, 99.65841279375145, 128.61923272576175, -124.45822725812972, 40.90493613558705, -133.24229002709237, 89.48386839465459, -88.73873161157177, 25.4987779561848, 139.30921989458596, -56.48047666665307, -54.42694931183609, 119.8132748415278, -43.00572569501252, 87.09611943074756, -132.94041310286832, -71.82144238108796, 50.6624159286875, 74.86938691787664, -106.22139160281148, 85.05101644182555, -121.33202375843675, -13.216691792290263, 147.74795828850577, -40.64082389519048, -2.293798744097962, 139.5443606212736, 19.705191808363946, -121.56147644234053, 176.17601104410812, 42.71119097543117, -160.8657949661788, 86.88855258158685, -24.19176463295591, 114.08803301389044, -124.09704835561679, -65.67062198302106, 14.22649077744474, 162.40073665232603, -55.8519752143678, 95.38880184677465, -141.4811606976856, -64.23565138209425, -22.796634850076533, 47.99159297343306, -161.5370251399869, 22.081842750096385, -61.41939135866188, 146.39069306042094, -22.85945608122077, -114.56094784553403, 70.96403766317401, -81.45755421519603, 136.33879997370917, -172.0768624725614, 18.12646423332207, -104.81760828295131, 80.86069891714214, -35.504076051150676, 166.814871502146, 28.714898182382967, -152.04073156583397, 44.63088930001562, 114.50939696489837, -35.9739711826192, -176.50915708556371, -50.44518909884993]} ("Phase spectrum"), "f0"=0.0, "df"=w7, "phase"=w40) -> (→"Phase spectrum":cluster{"f0":dbl, "df":dbl, "phase":dbl[]})
  n57 = Multiply(x=w68, y=20.0 ("f0")) -> (x*y=w67:dbl[])
  n58 = Bundle By Name(cluster=cluster{"f0":dbl, "df":dbl, "magnitude":dbl[]} {"f0"=0.0, "df"=0.0, "magnitude"=[]} ("Amplitude spectrum"), "f0"=0.0, "df"=w7, "magnitude"=w67) -> (→"Amplitude spectrum":cluster{"f0":dbl, "df":dbl, "magnitude":dbl[]})
